vi "UDP_Client.vi"() -> ()   [LabVIEW 2020]
uses:
  <vilib>/ErrorRing/Error Ring.xnode
panel:
  out "Waveform Chart":dbl(graph)
  out "data out":string
  in  "Puerto Destino":u16
  in  "String":string
  in  "stop":bool
  # "Cliente UDP Numero 1"
  # "Server UDP Numero 2"
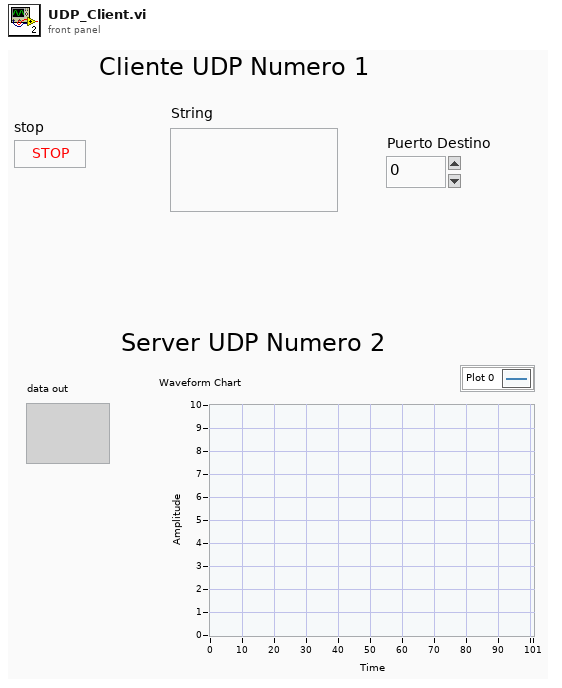
[diagram p1: front panel]
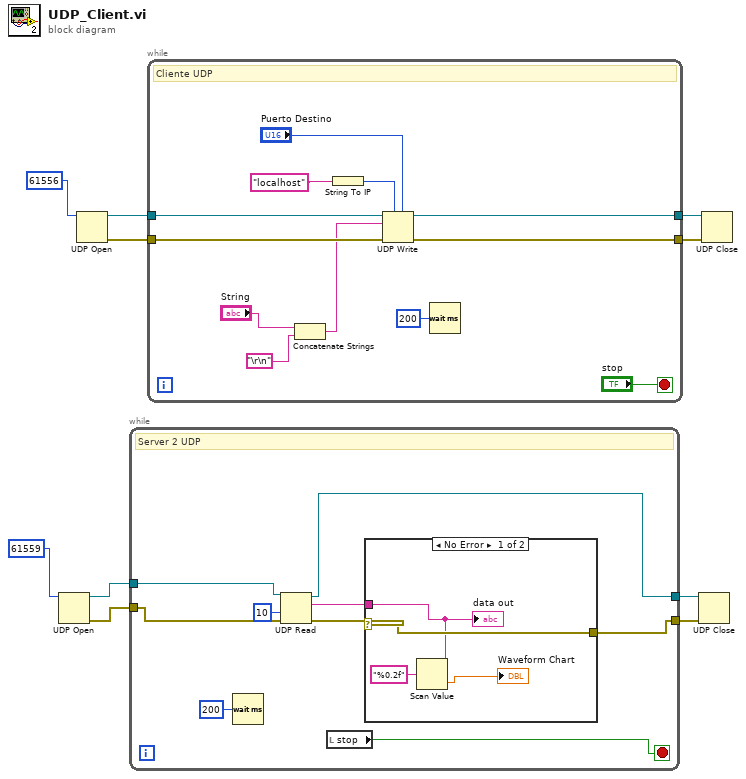
[diagram p0: block diagram]
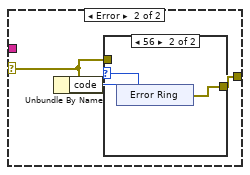
[diagram p2: hidden frame]
diagram:
  n1 = UDP Open(11:u16 61559 ("port")) -> (port=w4:refnum<k16>, 0:w5:errorcluster)  [unwired: 4 in, 1 out]
  n2 = UDP Open(11:u16 61556 ("port")) -> (port=w7:refnum<k16>, 0:w10:errorcluster)  [unwired: 4 in, 1 out]
  n3 = while {
    tunnel: w5 -> [w18]
    tunnel: w4 -> [w19]
    tunnel: [w15] -> w2
    tunnel: [w13] -> w1
    stop <- w12 stop-if-true
    # "Server 2 UDP"
    n4 = Wait (ms)(milliseconds to wait=u32 200) -> ()  [unwired: 1 out]
    n5 = UDP Read(connection ID=w19, timeout ms (25000)=10, 8:w18) -> (data out=w14:string, error out=w16:errorcluster, 3:w15:refnum<k16>)  [unwired: 1 in, 2 out]
    n6 = local read "stop"() -> (w12:bool)
    n7 = case shown="No Error" w16 {
      selector: w16 -> [w23 w24]
      tunnel: w14 -> [w22 _]
      tunnel: [w23 w25] -> w13
      frame No Error {
        n8 = Scan Value(string=w22, format string="%0.2f") -> (value=→"Waveform Chart":dbl)  [unwired: 1 in, 1 out]
        "data out" <- w22
      }
      frame Error {
        n9 = Unbundle By Name(w24) -> ("code"=w26:i32)
        n10 = case shown="56" w26 {
          tunnel: [w27 w28] -> w25
          tunnel: w24 -> [w27 _]
          frame 0, Default {
          }
          frame 56 {
            n11 = xnode "Error Ring"() -> ("error out"=w28:errorcluster)
          }
        }
      }
    }
  }
  n12 = while {
    tunnel: w10 -> [w40]
    tunnel: [w39] -> w9
    tunnel: [w38] -> w8
    tunnel: w7 -> [w37]
    stop <- "stop" stop-if-true
    # "Cliente UDP"
    n13 = Concatenate Strings("String", "\r\n") -> (w34:string)
    n14 = String To IP(1:"localhost" ("name")) -> (0:w33:u32)
    n15 = UDP Write(address=w33, port or service name="Puerto Destino", connection ID=w37, data in=w34, 8:w40) -> (error out=w39:errorcluster, 3:w38:refnum<k16>)  [unwired: 1 in]
    n16 = Wait (ms)(milliseconds to wait=u32 200) -> ()  [unwired: 1 out]
  }
  n17 = UDP Close(connection ID=w2, 8:w1) -> ()  [unwired: 2 out]
  n18 = UDP Close(connection ID=w8, 8:w9) -> ()  [unwired: 2 out]
